vi "Write retries.vi"(8 "error in (no error)":errorcluster, 10 "retries":i32=1, 11 "MB_Master_Serial in":refnum<class "MB_Master_Serial.lvclass">) -> (0 "error out":errorcluster, 3 "MB_Master_Serial out":refnum<class "MB_Master_Serial.lvclass">)   [LabVIEW 2016, in "MB Master.lvlib" / "MB_Master_Serial.lvclass"]
uses:
  MB_Master_Serial.lvclass
  MB_Master_Serial.lvclass/MB_Master_Serial.ctl
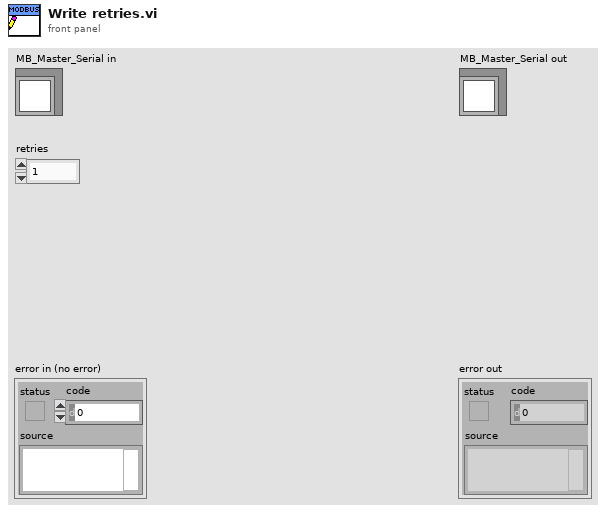
[diagram p1: front panel]
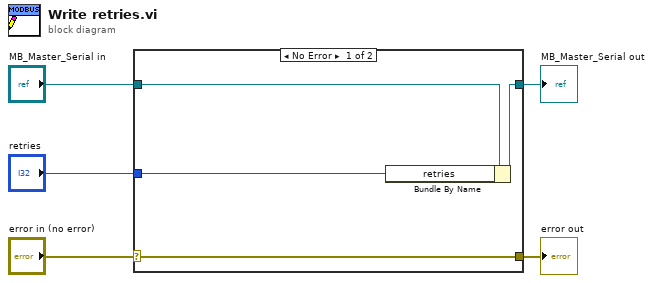
[diagram p0: block diagram]
diagram:
  n1 = case shown="No Error" "error in (no error)" {
    selector: "error in (no error)" -> [w9 w10]
    tunnel: [w9 w10] -> w4
    tunnel: [w7 w11] -> w2
    tunnel: "MB_Master_Serial in" -> [w8 w11]
    tunnel: "retries" -> [w6 _]
    frame No Error {
      n2 = Bundle By Name(cluster=w8, "retries"=w6) -> (w7:refnum<class "MB_Master_Serial.lvclass">)
    }
    frame Error {
    }
  }
  "error out" <- w4
  "MB_Master_Serial out" <- w2
